vi "Setup LED Array Interpolate.vi"(10 "Steps":i32, 11 "LEDs In":i32[][](array[numeric])) -> (3 "Interpolate Out":T1(array[cluster]))   [LabVIEW 2014]
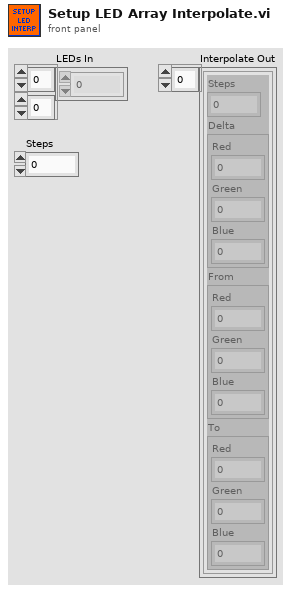
[diagram p1: front panel]
types:
  T1 = cluster{"Steps":i32, "Delta":cluster{"Red":dbl, "Green":dbl, "Blue":dbl}, "From":cluster{"Red":dbl, "Green":dbl, "Blue":dbl}, "To":cluster{"Red":dbl, "Green":dbl, "Blue":dbl}}[]
  T2 = cluster{"Steps":i32, "Delta":cluster{"Red":dbl, "Green":dbl, "Blue":dbl}, "From":cluster{"Red":dbl, "Green":dbl, "Blue":dbl}, "To":cluster{"Red":dbl, "Green":dbl, "Blue":dbl}}
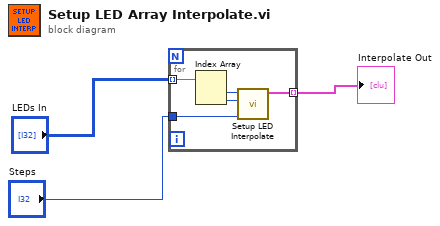
[diagram p0: block diagram]
diagram:
  n1 = for {
    tunnel: "LEDs In" -> [w8] mode=indexing
    tunnel: "Steps" -> [w5]
    tunnel: [w4] -> w3 mode=indexing
    n2 = Index Array(array=w8) -> (element #1=w7:i32, element #2=w6:i32)  [unwired: 2 in]
    n3 = call "Setup LED Interpolate.vi"("Steps"=w5, "To"=w6, "From"=w7) -> ("Cluster"=w4:T2)  [unwired: 8 in]
  }
  "Interpolate Out" <- w3
